vi "Update File Icon.vi"(0 "TreeControl in":refnum<vi>, 5 "Measurement file Tags":string[](array[string]), 7 "Folder Tag":string, 9 "Folder Icon":i32, 11 "error in (no error)":errorcluster) -> (4 "TreeControl out":refnum<vi>, 15 "error out":errorcluster)   [LabVIEW 2021, in "Converter.lvlib"]
uses:
  Converter.lvlib
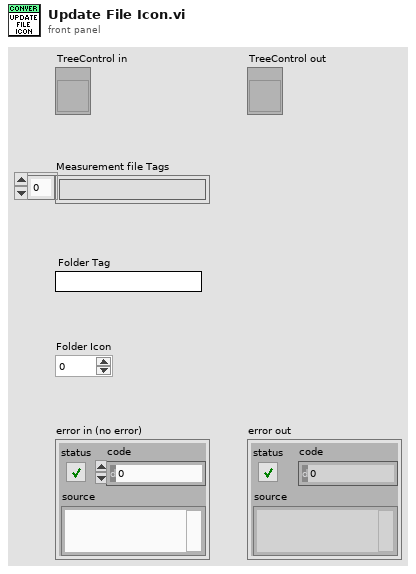
[diagram p1: front panel]
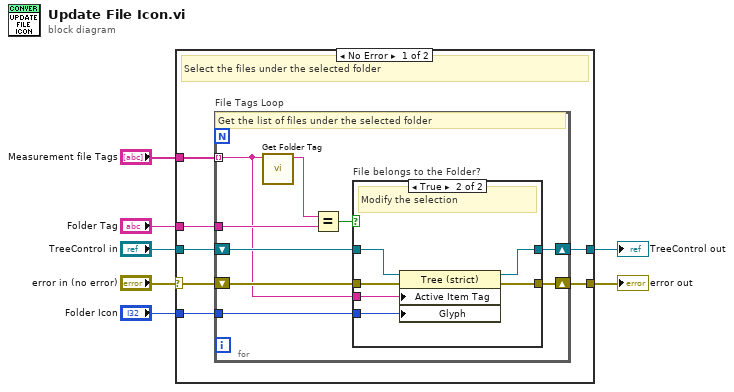
[diagram p0: block diagram]
diagram:
  n1 = case shown="No Error" "error in (no error)" {
    selector: "error in (no error)" -> [w9 w32]
    tunnel: [w14 w33] -> w7
    tunnel: [w13 w32] -> w6
    tunnel: "Folder Icon" -> [w12 _]
    tunnel: "TreeControl in" -> [w11 w33]
    tunnel: "Folder Tag" -> [w10 _]
    tunnel: "Measurement file Tags" -> [w8 _]
    frame No Error {
      # "Select the files under the selected folder"
      n2 = for "File Tags Loop" {
        tunnel: w8 -> [w16] mode=indexing
        tunnel: w10 -> [w18]
        shift-right: [w21] -> w13
        shift-left: w9 -> [w23]
        shift-right: [w19] -> w14
        shift-left: w11 -> [w20]
        tunnel: w12 -> [w22]
        # "Get the list of files under the selected folder"
        n3 = call "Get Folder Tag.vi"("Selected cell Tag"=w16) -> ("Folder Tag"=w15:string)  [unwired: 6 in]
        n4 = Equal?(x=w15, y=w18) -> (x = y?=w17:bool)
        n5 = case "File belongs to the Folder?" shown="True" w17 {
          tunnel: w23 -> [w25 w31]
          tunnel: w22 -> [_ w30]
          tunnel: [w25 w29] -> w21
          tunnel: w20 -> [w24 w28]
          tunnel: [w24 w27] -> w19
          tunnel: w16 -> [_ w26]
          frame False {
            # "Pass"
          }
          frame True {
            # "Modify the selection"
            n6 = property on="Property Node" class="Tree (strict)"(reference=w28, error in=w31, "Active Item Tag"=w26, "Glyph"=w30) -> (reference out=w27:refnum<vi>, error out=w29:errorcluster)
          }
        }
      }
    }
    frame Error {
      # "Pass"
    }
  }
  "TreeControl out" <- w7
  "error out" <- w6
